vi "Generate Package Integrity File.vi"(0 "PackageID":string, 1 "PackageRev":string, 2 "Purpose":string, 3 "System Key":string, 4 "USER_NAME":string, 5 "Error In":errorcluster, 6 "Package File Paths":path[](array[path]), 8 "Integrity File Path":path) -> (19 "error out":errorcluster)   [LabVIEW 2010]
doc: "This VI generates a Package Integrity File based on the parameters given to it.\n\nDan Woods\n7/2/02\nCopyright 2002 VI Engineering, Inc.\nCurrent Revision: 13\nVSS Version: 3"
uses:
  package/File Exists - Scalar__ogtk.vi
  <vilib>/Utility/config.llb/NI_LVConfig.lvlib
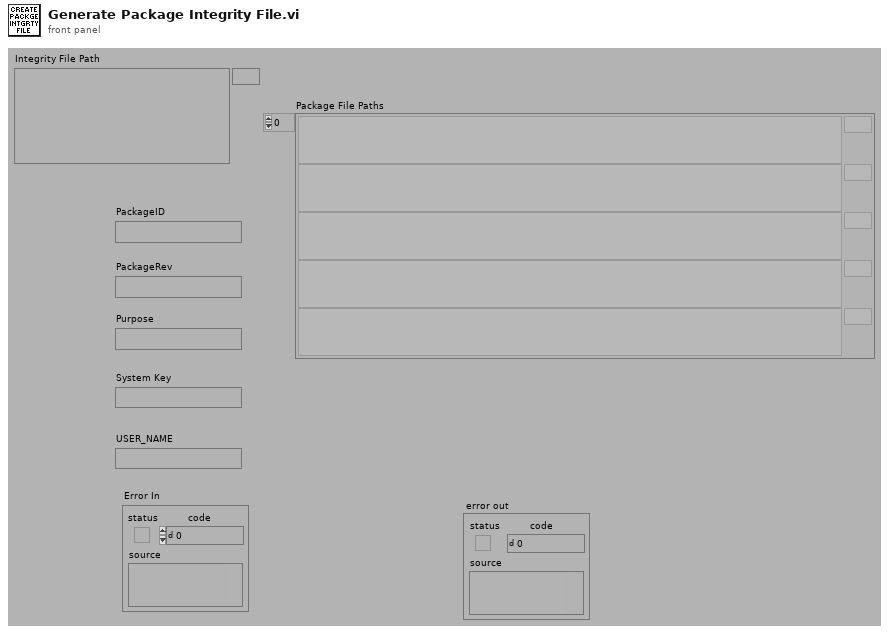
[diagram p1: front panel]
types:
  T1 = typedef "NI_LVConfig.lvlib/Config Data RefNum.ctl" = refnum<k1>
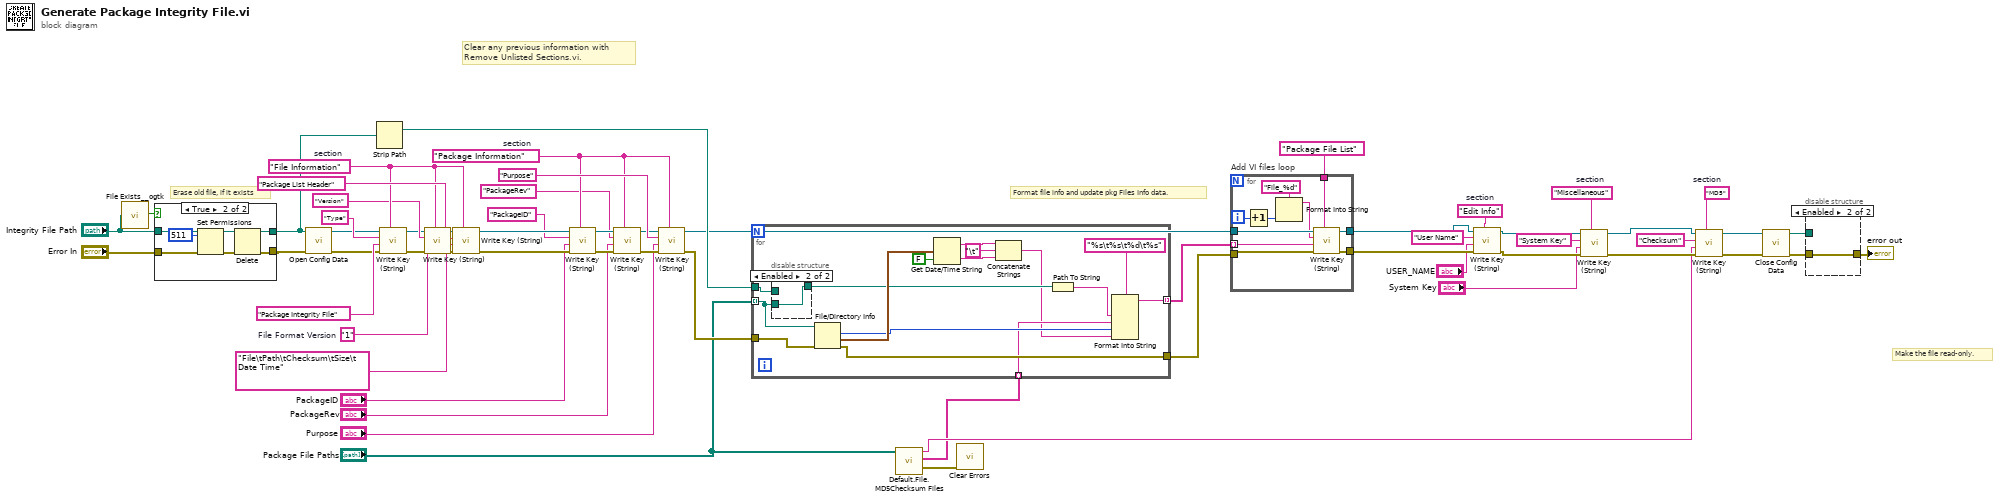
[diagram p0: block diagram]
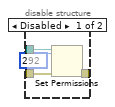
[diagram p2: hidden frame]
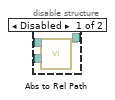
[diagram p4: hidden frame]
diagram:
  w8 = "MD5"  # section
  w18 = "Miscellaneous"  # section
  w19 = "Edit Info"  # section
  w59 = "Package Information"  # section
  w54 = "File Information"  # section
  w47 = "1"  # File Format Version
  # "Erase old file, if it exists"
  # "Make the file read-only."
  # "Format file info and update pkg Files Info data."
  # "Clear any previous information with Remove Unlisted Sections.vi."
  n1 = call-poly "File Exists__ogtk.vi"("file path"="Integrity File Path") -> ("exists"=w29:bool)  [unwired: 6 in, 1 out]
  n2 = case shown="True" w29 {
    tunnel: [w62 w68] -> w28
    tunnel: [w61 w65] -> w27
    tunnel: "Error In" -> [w61 w64]
    tunnel: "Integrity File Path" -> [w62 w63]
    frame False {
    }
    frame True {
      n3 = Set Permissions(7:i16 511 ("new permissions"), 8:w64, 11:w63) -> (0:w66:errorcluster, 3:w69:path)  [unwired: 2 in]
      n4 = Delete(path (use dialog)=w69, error in=w66) -> (deleted path=w68:path, error out=w65:errorcluster)  [unwired: 3 in, 1 out]
    }
  }
  n5 = call <vilib>:"Open Config Data.vi"("error in (no error)"=w27, "configuration file path"=w28) -> ("error out"=w25:errorcluster, "refnum"=w26:T1)  [unwired: 7 in, 1 out]
  n6 = Strip Path(path=w28) -> (stripped path=w32:path)  [unwired: 1 out]
  n7 = call <vilib>:"Write Key (String).vi"("section"=w54, "error in (no error)"=w25, "value"="Package Integrity File", "key"="Type", "refnum"=w26) -> ("error out"=w48:errorcluster, "refnum out"=w43:T1)  [unwired: 4 in, 1 out]
  n8 = call <vilib>:"Write Key (String).vi"("section"=w54, "error in (no error)"=w48, "value"=w47, "key"="Version", "refnum"=w43) -> ("error out"=w51:errorcluster, "refnum out"=w50:T1)  [unwired: 4 in, 1 out]
  n9 = call <vilib>:"Write Key (String).vi"("section"=w54, "error in (no error)"=w51, "value"="File\tPath\tChecksum\tSize\t Date Time", "key"="Package List Header", "refnum"=w50) -> ("error out"=w53:errorcluster, "refnum out"=w52:T1)  [unwired: 4 in, 1 out]
  n10 = call <vilib>:"Write Key (String).vi"("section"=w59, "error in (no error)"=w53, "value"="PackageID", "key"="PackageID", "refnum"=w52) -> ("error out"=w49:errorcluster, "refnum out"=w42:T1)  [unwired: 4 in, 1 out]
  n11 = call <vilib>:"Write Key (String).vi"("section"=w59, "error in (no error)"=w49, "value"="PackageRev", "key"="PackageRev", "refnum"=w42) -> ("error out"=w58:errorcluster, "refnum out"=w57:T1)  [unwired: 4 in, 1 out]
  n12 = call <vilib>:"Write Key (String).vi"("section"=w59, "error in (no error)"=w58, "value"="Purpose", "key"="Purpose", "refnum"=w57) -> ("error out"=w36:errorcluster, "refnum out"=w23:T1)  [unwired: 4 in, 1 out]
  n13 = call "Default.File.MD5Checksum Files.vi"("FilePaths"="Package File Paths") -> ("error out"=w2:errorcluster, "Checksum Array"=w1:string[], "MD5 message-digest"=w3:string)  [unwired: 8 in]
  n14 = for "VI Files Loop" {
    tunnel: "Package File Paths" -> [w73] mode=indexing
    tunnel: [w85] -> w34 mode=indexing
    tunnel: w32 -> [w83]
    tunnel: w36 -> [w79]
    tunnel: [w75] -> w24
    tunnel: w1 -> [w71] mode=indexing
    n15 = disable-structure shown="Enabled" {
      disable-tunnel: w83 -> [w88 _]
      disable-tunnel: [w87 w89] -> w74
      disable-tunnel: w73 -> [w86 w89]
      frame Disabled {
        n16 = call "Abs to Rel Path.vi"("File Path"=w86, "Base Path"=w88) -> ("Path Out"=w87:path)  [unwired: 8 in, 1 out]
      }
      frame Enabled {
      }
    }
    n17 = File/Directory Info(path=w73, error in=w79) -> (size=w72:i64, last mod=w80:timestamp, error out=w75:errorcluster)  [unwired: 4 out]
    n18 = Get Date/Time String(seconds (now)=w80, want seconds? (F)=FALSE) -> (date string=w77:string, time string=w78:string)  [unwired: 1 in]
    n19 = Concatenate Strings(w77, "\t" ("string"), w78) -> (w70:string)
    n20 = Path To String(path=w74) -> (string=w82:string)
    n21 = Format Into String(format string="%s\t%s\t%d\t%s" ("Format String"), w82, w71, w72, w70) -> (resulting string=w85:string)  [unwired: 2 in, 1 out]
  }
  n22 = call <vilib>:"Clear Errors.vi"("error in (no error)"=w2) -> ()  [unwired: 6 in, 1 out]
  n23 = for "Add VI files loop" {
    tunnel: w34 -> [w97] mode=indexing
    tunnel: w23 -> [w98]
    tunnel: "Package File List" ("section") -> [w99]
    tunnel: [w96] -> w14
    tunnel: w24 -> [w91]
    tunnel: [w90] -> w13
    i -> [w93]
    n24 = Increment(x=w93) -> (x+1=w92:i32)
    n25 = Format Into String(format string="File_%d" ("Format String"), w92) -> (resulting string=w94:string)  [unwired: 2 in, 1 out]
    n26 = call <vilib>:"Write Key (String).vi"("section"=w99, "error in (no error)"=w91, "value"=w97, "key"=w94, "refnum"=w98) -> ("error out"=w96:errorcluster, "refnum out"=w90:T1)  [unwired: 4 in, 1 out]
  }
  n27 = call <vilib>:"Write Key (String).vi"("section"=w19, "error in (no error)"=w14, "value"="USER_NAME", "key"="User Name", "refnum"=w13) -> ("error out"=w15:errorcluster, "refnum out"=w16:T1)  [unwired: 4 in, 1 out]
  n28 = call <vilib>:"Write Key (String).vi"("section"=w18, "error in (no error)"=w15, "value"="System Key", "key"="System Key", "refnum"=w16) -> ("error out"=w5:errorcluster, "refnum out"=w6:T1)  [unwired: 4 in, 1 out]
  n29 = call <vilib>:"Write Key (String).vi"("section"=w8, "error in (no error)"=w5, "value"=w3, "key"="Checksum", "refnum"=w6) -> ("error out"=w4:errorcluster, "refnum out"=w7:T1)  [unwired: 4 in, 1 out]
  n30 = call <vilib>:"Close Config Data.vi"("error in (no error)"=w4, "refnum"=w7) -> ("error out"=w22:errorcluster, "file path"=w21:path)  [unwired: 8 in]
  n31 = disable-structure shown="Enabled" {
    disable-tunnel: [w102 w104] -> w33
    disable-tunnel: w22 -> [w101 w104]
    disable-tunnel: w21 -> [w100 _]
    frame Disabled {
      n32 = Set Permissions(7:i16 292 ("new permissions"), 8:w101, 11:w100) -> (0:w102:errorcluster)  [unwired: 2 in, 1 out]
    }
    frame Enabled {
    }
  }
  "error out" <- w33
